vi "Write Element of Values.vi"(9 "Variant":variant, 10 "indices":i32[](array[numeric]), 11 "Series in":refnum<class "Series.lvclass">) -> (3 "Series out":refnum<class "Series.lvclass">)   [LabVIEW 2017]
uses:
  Series.lvclass
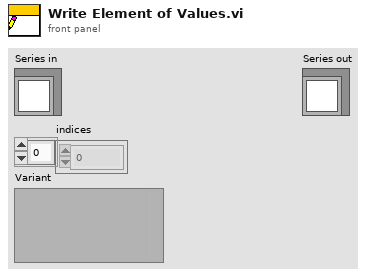
[diagram p1: front panel]
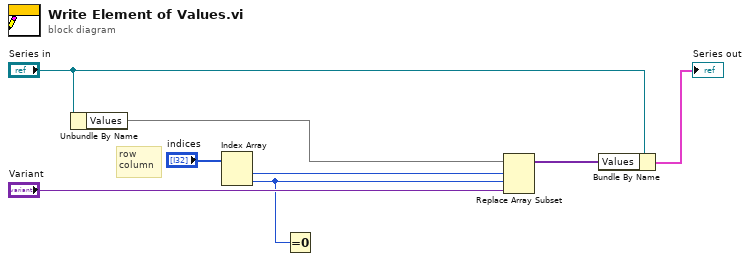
[diagram p0: block diagram]
diagram:
  # "row\ncolumn"
  n1 = Unbundle By Name("Series in") -> ("Values"=w1)
  n2 = Index Array(array="indices") -> (element #1=w3:i32, element #2=w2:i32)  [unwired: 2 in]
  n3 = Equal To 0?(x=w2) -> ()  [unwired: 1 out]
  n4 = Replace Array Subset(array=w1, new element="Variant", index (row)=w3, index (col)=w2) -> (w5:variant[])
  n5 = Bundle By Name(cluster="Series in", "Values"=w5) -> (→"Series out":cluster{})
